vi "Read Components Ref.vi"(8 "error in (no error)":errorcluster, 11 "Item Ref in":T1 format="%.0x") -> (0 "error out":errorcluster, 2 "Components":refnum<class "Component.lvclass">[](array[class]), 3 "Item Ref out":T1 format="%.0x")   [LabVIEW 2020, in "DSF System Explorer.lvlib"]
uses:
  DSF System Explorer.lvlib
  <vilib>/NI VeriStand/Custom Device API/Custom Device Item Ref.ctl
  DSF Core.lvlibp/Classes/Component/Component.lvclass
  <vilib>/NI VeriStand/Custom Device API/Custom Device API.lvlib
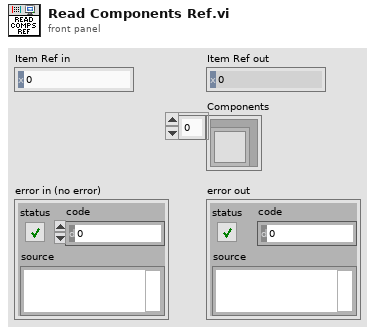
[diagram p1: front panel]
types:
  T1 = typedef "Custom Device API.lvlib/Custom Device Item Ref.ctl" = u64
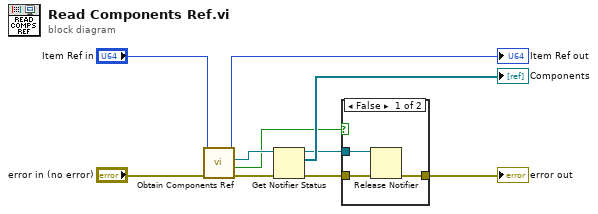
[diagram p0: block diagram]
diagram:
  n1 = call "Obtain Components Ref.vi"("error in (no error)"="error in (no error)", "Item Ref in"="Item Ref in") -> ("error out"=w2:errorcluster, "created new?"=w1:bool, "comps notifier"=w4:refnum<notifier>, "Item Ref out"=→"Item Ref out":T1)  [unwired: 6 in]
  n2 = Get Notifier Status(notifier=w4, error in (no error)=w2) -> (notifier out=w3:refnum<notifier>, current notification=→"Components":refnum<class "Component.lvclass">[], error out=w5:errorcluster)  [unwired: 2 out]
  n3 = case shown="False" w1 {
    tunnel: w5 -> [w13 w14]
    tunnel: w3 -> [w12 _]
    tunnel: [w11 w14] -> w9
    frame False {
      n4 = Release Notifier(notifier=w12, error in (no error)=w13) -> (error out=w11:errorcluster)  [unwired: 1 in, 2 out]
    }
    frame True {
    }
  }
  "error out" <- w9
